vi "XML Script - Constant (Variant).vi"(0 "x":i32=-1, 1 "y":i32=-1, 2 "out":i32=-1, 4 "typeindex":i32=-1, 6 "name":string, 8 "vi path":path, 9 "prefix (name)":string, 10 "in":i32=-1) -> (5 "name (wire source)":string, 7 "XML Script Command - Constant (I32)":string)   [LabVIEW 2020]
uses:
  <vilib>/_script/XML Scripting/XML Script Tag.ctl
  <vilib>/_script/XML Scripting/XML Script Attribute.ctl
  <vilib>/_script/XML Scripting/XML Script - PathToXMLString.vi
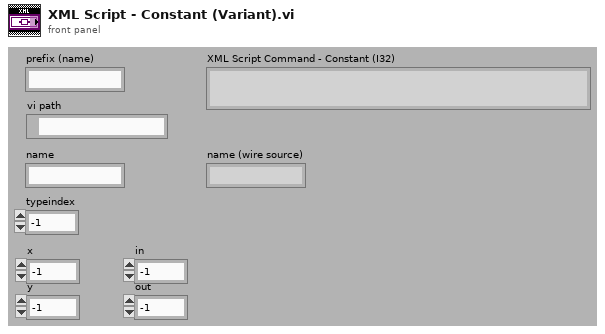
[diagram p1: front panel]
types:
  T1 = typedef "XML Script Attribute.ctl" = enum16{"name", "style", "path", "position", "in", "out", "width", "height", "index", "value", "default", "location", "offset", "typeindex", "size", "source", "destination", "indicator", "type", "controlname", "label", "conpaneidx", "mode", "description", "hasCondTerm", "linkIdentity", "caseselectortype", "concatInputs", "inName", "instantiationpath", "loopCondition", "IndexMode", "formulaInputs", "formulaOutputs", "msnFuncName", "msnIsDynamic", "msnIsODEUserFunction", "ignoreSearchDialog"}
  T2 = typedef "XML Script Tag.ctl" = enum16{"Script", "Function", "SubVI", "GrowableFunction", "Structure", "MultiframeStructure", "Frame", "Tunnel", "ShiftRegister", "Constant", "Control", "Terminal", "Wire", "StaticVIReference", "ControlTerminal", "CompoundArithmetic", "FlatSequence", "FlatSequenceFrame", "MathScriptCallByRef", "BuildArray", "GenericSubVI", "MathScriptNode"}
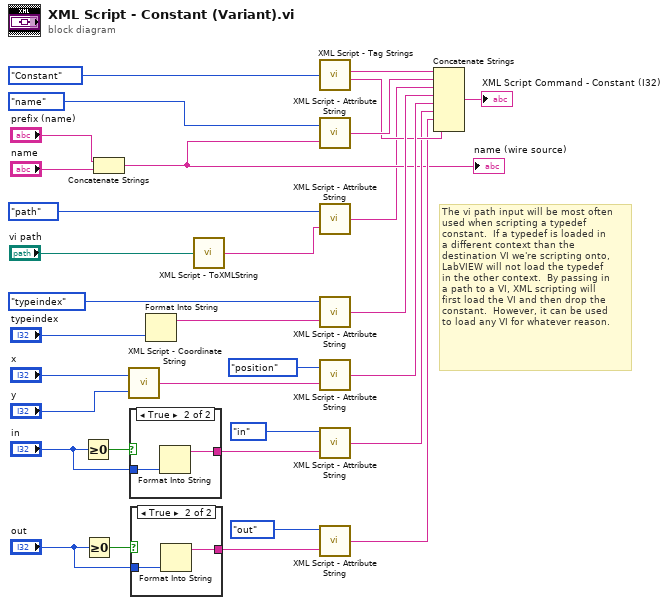
[diagram p0: block diagram]
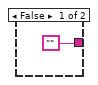
[diagram p2: hidden frame]
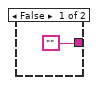
[diagram p3: hidden frame]
diagram:
  # "The vi path input will be most often\nused when scripting a typedef\nconstant.  If a typedef is loaded in\na different context than the\ndestination VI we're scripting onto,\nLabVIEW will not load the typedef\nin the other context.  By passing in\na path to a VI, XML scripting will\nfirst load the VI and then drop the\nconstant.  However, it can be used\nto load any VI for whatever reason."
  n1 = Greater Or Equal To 0?(x="in") -> (x >= 0?=w14:bool)
  n2 = Greater Or Equal To 0?(x="out") -> (x >= 0?=w18:bool)
  n3 = Concatenate Strings("prefix (name)", "name") -> (w7:string)
  "name (wire source)" <- w7
  n4 = call <vilib>:"XML Script - Coordinate String.vi"("y"="y", "x"="x") -> ("(x,y)"=w23:string)
  n5 = case shown="True" w14 {
    tunnel: "in" -> [_ w35]
    tunnel: ["" w34] -> w16
    frame False {
    }
    frame True {
      n6 = Format Into String(w35) -> (resulting string=w34:string)  [unwired: 3 in, 1 out]
    }
  }
  n7 = case shown="True" w18 {
    tunnel: "out" -> [_ w38]
    tunnel: ["" w37] -> w20
    frame False {
    }
    frame True {
      n8 = Format Into String(w38) -> (resulting string=w37:string)  [unwired: 3 in, 1 out]
    }
  }
  n9 = Format Into String("typeindex") -> (resulting string=w5:string)  [unwired: 3 in, 1 out]
  n10 = call-poly <vilib>:"XML Script - ToXMLString.vi"("Path"="vi path") -> ("Valid XML String (out)"=w1:string)
  n11 = call <vilib>:"XML Script - Tag Strings.vi"("XML Script Tag"=XML_Script_Tag."Constant") -> ("XML String - Begin Tag"=w28:string, "XML String - End Tag"=w12:string)  [unwired: 2 in]
  n12 = call <vilib>:"XML Script - Attribute String.vi"("Attribute String"=w7, "XML Script Attribute"=XML_Script_Attribute."name") -> ("XML Script - Attribute String"=w26:string)
  n13 = call <vilib>:"XML Script - Attribute String.vi"("Attribute String"=w1, "XML Script Attribute"=XML_Script_Attribute."path") -> ("XML Script - Attribute String"=w3:string)
  n14 = call <vilib>:"XML Script - Attribute String.vi"("Attribute String"=w5, "XML Script Attribute"=XML_Script_Attribute."typeindex") -> ("XML Script - Attribute String"=w24:string)
  n15 = call <vilib>:"XML Script - Attribute String.vi"("Attribute String"=w23, "XML Script Attribute"=XML_Script_Attribute."position") -> ("XML Script - Attribute String"=w22:string)
  n16 = call <vilib>:"XML Script - Attribute String.vi"("Attribute String"=w16, "XML Script Attribute"=XML_Script_Attribute."in") -> ("XML Script - Attribute String"=w10:string)
  n17 = call <vilib>:"XML Script - Attribute String.vi"("Attribute String"=w20, "XML Script Attribute"=XML_Script_Attribute."out") -> ("XML Script - Attribute String"=w11:string)
  n18 = Concatenate Strings(w28, w26, w3, w24, w22, w10, w11, w12) -> (→"XML Script Command - Constant (I32)":string)
